vi "Get All Environment Variables [Arrays].vi"(7 "Target (Process)":T1 items=["Process", "User", "Machine"], 8 "Error In":errorcluster) -> (0 "Error Out":errorcluster, 2 "Values[]":string[](array[string]), 3 "Names[]":string[](array[string]))   [LabVIEW 2023, in "SLL Environment Variable.lvlib"]
doc: "Retrieve all environment variables and their values from the target environment."
uses:
  SLL Environment Variable.lvlib
  _Typedef/Target Environment Enum.ctl
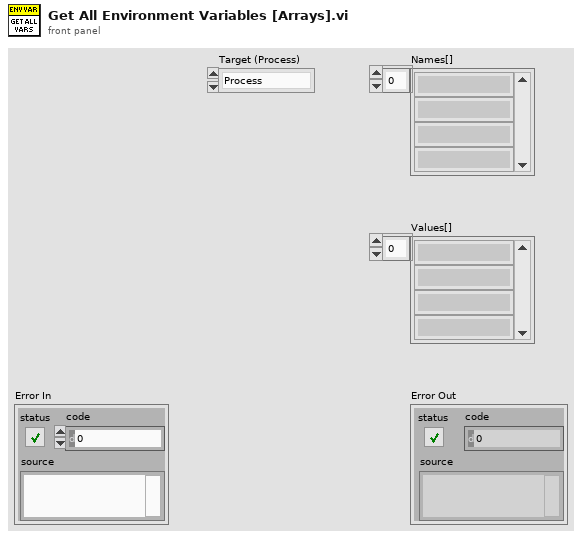
[diagram p1: front panel]
types:
  T1 = typedef "SLL Environment Variable.lvlib/Target Environment Enum.ctl" = i32
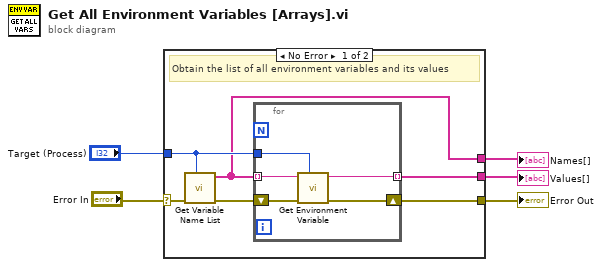
[diagram p0: block diagram]
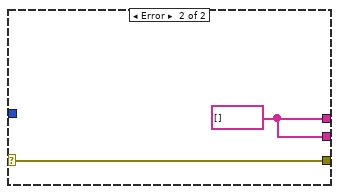
[diagram p2: hidden frame]
diagram:
  n1 = case shown="No Error" "Error In" {
    selector: "Error In" -> [w11 w18]
    tunnel: [w9 w18] -> w5
    tunnel: "Target (Process)" -> [w8 _]
    tunnel: [w7 w17] -> w2
    tunnel: [w6 w17] -> w1
    frame No Error {
      # "Obtain the list of all environment variables and its values"
      n2 = call "Get Variable Name List.vi"("Target (Process)"=w8, "Error In"=w11) -> ("Error Out"=w10:errorcluster, "Names[]"=w6:string[])  [unwired: 8 in]
      n3 = for {
        shift-right: [w15] -> w9
        shift-left: w10 -> [w16]
        tunnel: w6 -> [w14] mode=indexing
        tunnel: w8 -> [w13]
        tunnel: [w12] -> w7 mode=indexing
        n4 = call "Get Environment Variable.vi"("Target (Process)"=w13, "Error In"=w16, "Name"=w14) -> ("Error Out"=w15:errorcluster, "Value"=w12:string)  [unwired: 7 in]
      }
    }
    frame Error {
      w17 = string[] [] ("Names[]")
    }
  }
  "Error Out" <- w5
  "Values[]" <- w2
  "Names[]" <- w1
